vi "insert channel.vi"(8 "number of available channels":u16, 9 "Volts":T1={"conversion matrix"=[[0.0, 0.0], [0.0, 0.0], [0.0, 0.0], [0.0, 0.0], [0.0, 0.0], [0.0, 0.0]], "units"="volts", "name"="", "scale type"=enum."Volts", "offset (volts)"=0.0, "second channel"=0, "correspondence table"=[], "offset (physical units)"=0.0, "pH scale"={"Buffers"=[], "Temperature"=0.0}, "D.O."={"Temperature"=0.0, "K"=0.0, "barometric pressure"=0.0}} {"D.O."."K" format="%.6f"; "D.O."."Temperature" format="%.2f"; "pH scale"."Buffers"."V/T" format="%.5f"; "pH scale"."Buffers"."Buffer" format="%.2f"; "pH scale"."Temperature" format="%.2f"; "offset (physical units)" format="%.5f"; "correspondence table"."volts" format="%.4f"; "correspondence table"."physical units" format="%.4f"; "second channel" min=-1; "offset (volts)" format="%.5f"; "conversion matrix" format="%.4e"}, 10 "Sensor Array":T6, 11 "Index":u32) -> (2 "Sensor Array out":T6, 3 "Index out":u32)   [LabVIEW 2012]
uses:
  DAQ configuration/Sensor array.ctl
  DAQ configuration/channel identifier.ctl
  conversion.ctl
  DAQ configuration/scale type.ctl
  correspondence table.ctl
  pH/pH scale.ctl
  Dissolved Oxygen/DO scale.ctl
  global scale array.vi
panel:
  # "C"
  # "kPa"
  # "C"
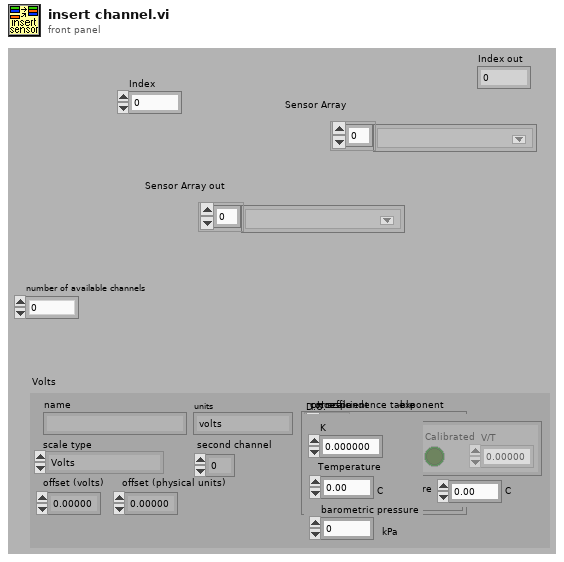
[diagram p1: front panel]
types:
  T1 = typedef "conversion.ctl" = cluster{"conversion matrix":sgl[][], "units":string, "name":string, "scale type":T2, "offset (volts)":dbl, "second channel":i8, "correspondence table":T3, "offset (physical units)":dbl, "pH scale":T4, "D.O.":T5}
  T2 = typedef "scale type.ctl" = enum16{"Volts", "Polynomial", "Correspondence Table", "pH", "Dissolved Oxygen", "Quadratic"}
  T3 = typedef "correspondence table.ctl" = cluster{"physical units":dbl, "volts":dbl}[]
  T4 = typedef "pH scale.ctl" = cluster{"Buffers":cluster{"Buffer":dbl, "Calibrated":bool, "V/T":dbl}[], "Temperature":dbl}
  T5 = typedef "DO scale.ctl" = cluster{"Temperature":dbl, "K":dbl, "barometric pressure":dbl}
  T6 = typedef "Sensor array.ctl" = T7[]
  T7 = typedef "channel identifier.ctl" = u16
  T8 = typedef "calib array.ctl" = T1[]
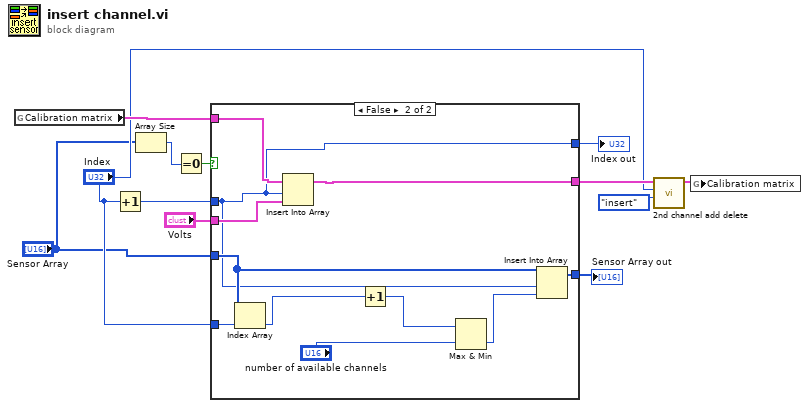
[diagram p0: block diagram]
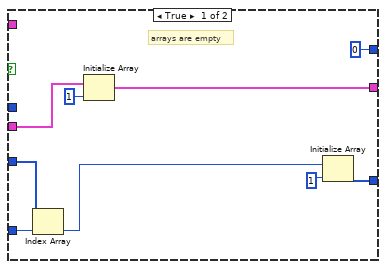
[diagram p2: hidden frame]
diagram:
  n1 = global read "global scale array.vi" "Calibration matrix"() -> (w11:T8)
  n2 = Increment(x="Index") -> (x+1=w12:u32)
  n3 = Array Size(array="Sensor Array") -> (size(s)=w10:i32)
  n4 = Equal To 0?(x=w10) -> (x = 0?=w9:bool)
  n5 = case shown="False" w9 {
    tunnel: "Index" -> [w21 w32]
    tunnel: w12 -> [_ w26]
    tunnel: w11 -> [_ w31]
    tunnel: "Sensor Array" -> [w16 w30]
    tunnel: [w15 w29] -> w8
    tunnel: [w19 w28] -> w5
    tunnel: "Volts" -> [w20 w27]
    tunnel: [u32 0 ("Index out") w26] -> w6
    frame True {
      # "arrays are empty"
      n6 = Index Array(array=w16, index=w21) -> (element=w13:T7)
      n7 = Initialize Array(w20, 1 ("Dimension Size")) -> (w19:T1[])
      n8 = Initialize Array(w13, 1 ("Dimension Size")) -> (w15:T7[])
    }
    frame False {
      n9 = Index Array(array=w30, index=w32) -> (element=w25:T7)
      n10 = Insert Into Array(array=w31, index=w26, new element=w27) -> (w28:T8)
      n11 = Increment(x=w25) -> (x+1=w23:T7)
      n12 = Max & Min(x=w23, y="number of available channels") -> (min(x,y)=w22:T7)  [unwired: 1 out]
      n13 = Insert Into Array(array=w30, index=w26, new element=w22) -> (w29:T6)
    }
  }
  "Sensor Array out" <- w8
  "Index out" <- w6
  n14 = call "2nd channel add delete.vi"("action"=enum16{"delete", "insert"}."insert", "Index"="Index", "Calibration array"=w5) -> ("Calibration array out"=w2:T8)  [unwired: 8 in]
  n15 = global write "global scale array.vi" "Calibration matrix"(w2) -> ()
